vi "SW_Set_Add_Recording_Settings.vi"(2 "Offsets, swaps and rotations in":T1={"Offset V."=0.0, "Offset H."=0.0, "Bridge swap"=FALSE, "Twisted neck"=FALSE, "Name prefix"="SavedTrack", "Stop at"=0.0, "\"Stop at\" enabled"=FALSE} {"Stop at" min=0.0 max=43200.0 step=60.0 format="%<%H:%M:%S>t"}) -> (0 "Offsets, swaps and rotations out":T1={"Offset V."=0.0, "Offset H."=0.0, "Bridge swap"=FALSE, "Twisted neck"=FALSE, "Name prefix"="SavedTrack", "Stop at"=0.0, "\"Stop at\" enabled"=FALSE} {"Stop at" min=0.0 max=43200.0 step=60.0 format="%<%H:%M:%S>t"})   [LabVIEW 2016]
uses:
  <vilib>/Utility/miscctls.llb/LVPointTypeDef.ctl
panel:
  out "\"Stop at\" buffer":dbl min=0.0 max=43200.0 step=60.0 format="%<%H:%M:%S>t"
  in  "Enable":bool
  in  "Bridge hor. offset":sgl min=-70 max=70 step=0.1 format="%#.1g"
  in  "Bridge swap":bool
  in  "Bridge offset":sgl min=-70 max=70 step=0.1 format="%#.1g"
  in  "Twisted neck":bool
  in  "Name Prefix":string="SavedTrack"
  in  "Stop record at":dbl=600.0 caption="Stop at" min=0.0 max=43200.0 step=60.0 format="%<%H:%M:%S>t"
  in  "Reset to defaults":bool
  in  "Exit":bool
  in  "Save Config":bool
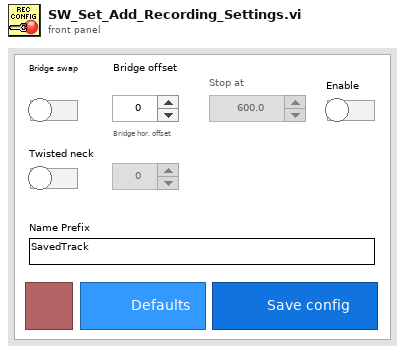
[diagram p1: front panel]
types:
  T1 = cluster{"Offset V.":sgl, "Offset H.":sgl, "Bridge swap":bool, "Twisted neck":bool, "Name prefix":string, "Stop at":dbl, "\"Stop at\" enabled":bool}
  T2 = typedef "LVPointTypeDef.ctl" = cluster{"Horizontal":i16, "Vertical":i16}
  T3 = enum8{"Enabled", "Disabled", "Disabled and Grayed Out"}
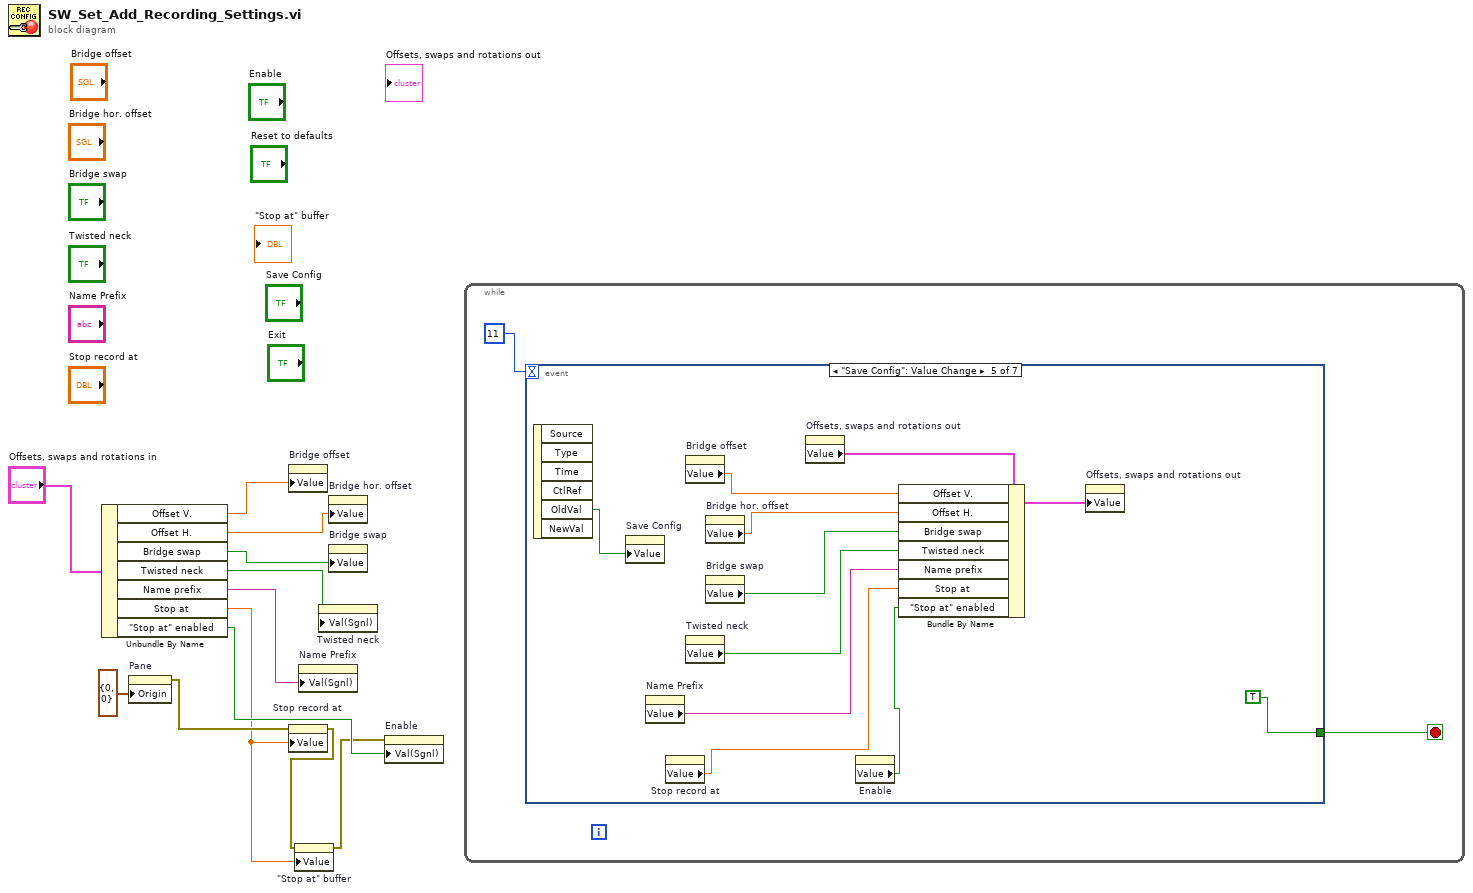
[diagram p0: block diagram]
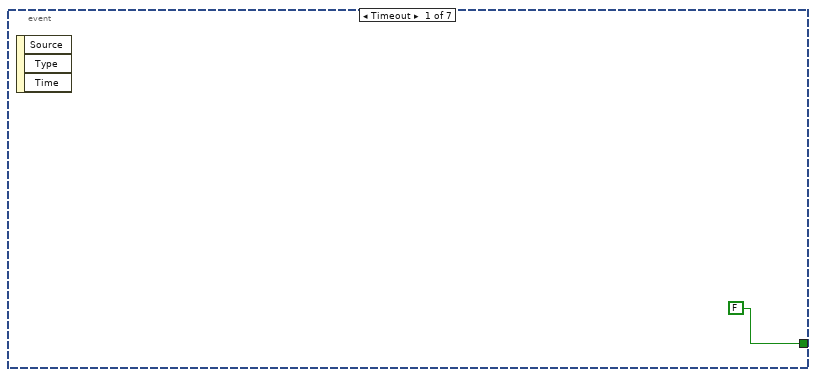
[diagram p2: hidden frame]
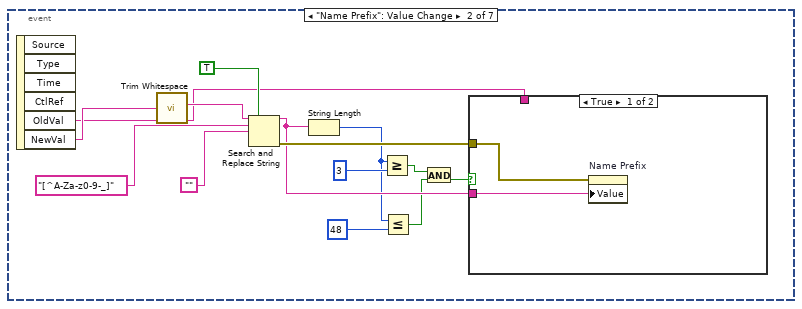
[diagram p3: hidden frame]
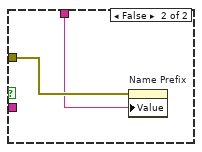
[diagram p4: hidden frame]
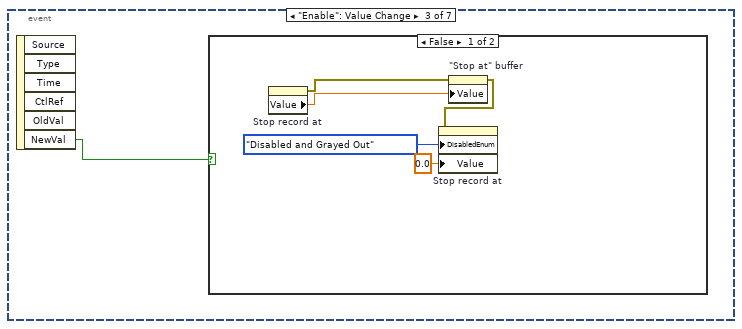
[diagram p5: hidden frame]
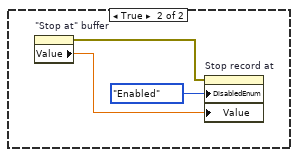
[diagram p6: hidden frame]
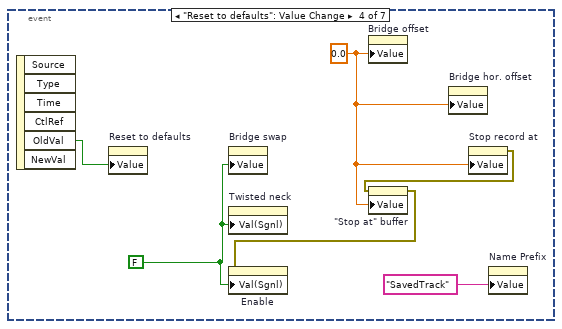
[diagram p7: hidden frame]
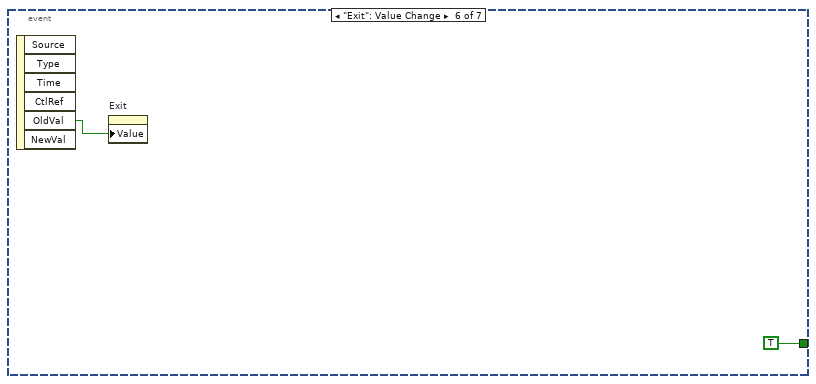
[diagram p8: hidden frame]
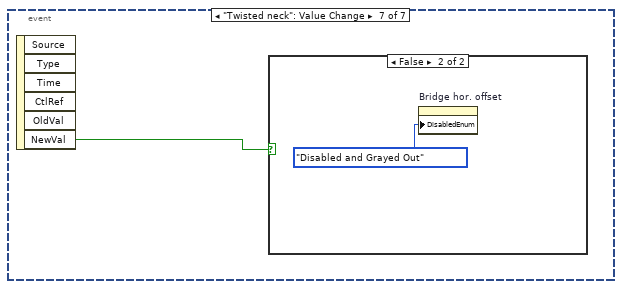
[diagram p9: hidden frame]
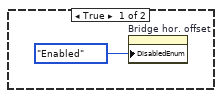
[diagram p10: hidden frame]
diagram:
  n1 = Unbundle By Name("Offsets, swaps and rotations in") -> ("Offset V."=w10:sgl, "Offset H."=w9:sgl, "Bridge swap"=w8:bool, "Twisted neck"=w7:bool, "Name prefix"=w6:string, "Stop at"=w1:dbl, "\"Stop at\" enabled"=w4:bool)
  n2 = property on="Pane" class="Pane"("Origin"=T2 {"Horizontal"=0, "Vertical"=0}) -> (error out=w5:errorcluster)  [unwired: 2 in, 1 out]
  n3 = property on="Bridge offset" class="DigNum (strict)"("Value"=w10) -> ()  [unwired: 2 in, 2 out]
  n4 = property on="Stop record at" class="DigNum (strict)"(error in=w5, "Value"=w1) -> (error out=w3:errorcluster)  [unwired: 1 in, 1 out]
  n5 = property on="\"Stop at\" buffer" class="DigNum (strict)"(error in=w3, "Value"=w1) -> (error out=w2:errorcluster)  [unwired: 1 in, 1 out]
  n6 = property on="Name Prefix" class="Str"("Val(Sgnl)"=w6) -> ()  [unwired: 2 in, 2 out]
  n7 = property on="Twisted neck" class="Bool (strict)"("Val(Sgnl)"=w7) -> ()  [unwired: 2 in, 2 out]
  n8 = property on="Bridge hor. offset" class="DigNum (strict)"("Value"=w9) -> ()  [unwired: 2 in, 2 out]
  n9 = property on="Bridge swap" class="Bool (strict)"("Value"=w8) -> ()  [unwired: 2 in, 2 out]
  n10 = property on="Enable" class="Bool (strict)"(error in=w2, "Val(Sgnl)"=w4) -> ()  [unwired: 1 in, 2 out]
  n11 = while {
    stop <- w13 stop-if-true
    n12 = event shown="[4] \"Save Config\": Value Change" {
      selector: _ -> [_ _ _ _ _ _ _]
      dyn-events: _ -> [_ _ _ _ _ _ _]
      timeout: 11 -> [_ _ _ _ _ _ _]
      tunnel: [FALSE _ _ _ TRUE TRUE _] -> w13
      event Timeout {
        n13 = event-data() -> ()  [unwired: 1 in, 3 out]
      }
      event "Name Prefix": Value Change {
        n14 = event-data() -> ("OldVal"=w20:string, "NewVal"=w21:string)  [unwired: 1 in, 4 out]
        n15 = call <vilib>:"Trim Whitespace.vi"("string"=w21) -> ("trimmed string"=w27:string)  [unwired: 1 in]
        n16 = Search and Replace String(replace all?=TRUE ("replace all? (F)"), input string=w27, search string="[^A-Za-z0-9-_]" ("regular expression"), replace string="") -> (result string=w22:string, error out=w24:errorcluster)  [unwired: 4 in, 2 out]
        n17 = String Length(string=w22) -> (length=w19:i32)
        n18 = Greater Or Equal?(x=w19, y=3) -> (x >= y?=w23:bool)
        n19 = Less Or Equal?(x=w19, y=48) -> (x <= y?=w16:bool)
        n20 = And(x=w23, y=w16) -> (x .and. y?=w17:bool)
        n21 = case shown="True" w17 {
          tunnel: w24 -> [w31 w33]
          tunnel: w22 -> [w30 _]
          tunnel: w20 -> [_ w32]
          frame True {
            n22 = property on="Name Prefix" class="Str"(error in=w31, "Value"=w30) -> ()  [unwired: 1 in, 2 out]
          }
          frame False {
            n23 = property on="Name Prefix" class="Str"(error in=w33, "Value"=w32) -> ()  [unwired: 1 in, 2 out]
          }
        }
      }
      event "Enable": Value Change {
        n24 = event-data() -> ("NewVal"=w34:bool)  [unwired: 1 in, 5 out]
        n25 = case shown="False" w34 {
          frame False {
            n26 = property on="Stop record at" class="DigNum (strict)"() -> (error out=w36:errorcluster, "Value"=w37:dbl)  [unwired: 2 in, 1 out]
            n27 = property on="\"Stop at\" buffer" class="DigNum (strict)"(error in=w36, "Value"=w37) -> (error out=w35:errorcluster)  [unwired: 1 in, 1 out]
            n28 = property on="Stop record at" class="DigNum (strict)"(error in=w35, "DisabledEnum"=T3."Disabled and Grayed Out" ("Disabled"), "Value"=0.0 ("Stop record at")) -> ()  [unwired: 1 in, 2 out]
          }
          frame True {
            n29 = property on="\"Stop at\" buffer" class="DigNum (strict)"() -> (error out=w40:errorcluster, "Value"=w41:dbl)  [unwired: 2 in, 1 out]
            n30 = property on="Stop record at" class="DigNum (strict)"(error in=w40, "DisabledEnum"=T3."Enabled" ("Disabled"), "Value"=w41) -> ()  [unwired: 1 in, 2 out]
          }
        }
      }
      event "Reset to defaults": Value Change {
        w45 = sgl 0.0 ("Bridge offset")
        w47 = FALSE
        n31 = event-data() -> ("OldVal"=w48:bool)  [unwired: 1 in, 5 out]
        n32 = property on="Reset to defaults" class="Bool (strict)"("Value"=w48) -> ()  [unwired: 2 in, 2 out]
        n33 = property on="Bridge swap" class="Bool (strict)"("Value"=w47) -> ()  [unwired: 2 in, 2 out]
        n34 = property on="Twisted neck" class="Bool (strict)"("Val(Sgnl)"=w47) -> ()  [unwired: 2 in, 2 out]
        n35 = property on="Bridge offset" class="DigNum (strict)"("Value"=w45) -> ()  [unwired: 2 in, 2 out]
        n36 = property on="Bridge hor. offset" class="DigNum (strict)"("Value"=w45) -> ()  [unwired: 2 in, 2 out]
        n37 = property on="Stop record at" class="DigNum (strict)"("Value"=w45) -> (error out=w44:errorcluster)  [unwired: 2 in, 1 out]
        n38 = property on="\"Stop at\" buffer" class="DigNum (strict)"(error in=w44, "Value"=w45) -> (error out=w43:errorcluster)  [unwired: 1 in, 1 out]
        n39 = property on="Enable" class="Bool (strict)"(error in=w43, "Val(Sgnl)"=w47) -> ()  [unwired: 1 in, 2 out]
        n40 = property on="Name Prefix" class="Str"("Value"="SavedTrack" ("Value (Signaling)")) -> ()  [unwired: 2 in, 2 out]
      }
      event "Save Config": Value Change {
        n41 = event-data() -> ("OldVal"=w56:bool)  [unwired: 1 in, 5 out]
        n42 = property on="Save Config" class="Bool (strict)"("Value"=w56) -> ()  [unwired: 2 in, 2 out]
        n43 = property on="Name Prefix" class="Str"() -> ("Value"=w51:string)  [unwired: 2 in, 2 out]
        n44 = property on="Stop record at" class="DigNum (strict)"() -> ("Value"=w50:dbl)  [unwired: 2 in, 2 out]
        n45 = property on="Bridge offset" class="DigNum (strict)"() -> ("Value"=w55:sgl)  [unwired: 2 in, 2 out]
        n46 = property on="Twisted neck" class="Bool (strict)"() -> ("Value"=w52:bool)  [unwired: 2 in, 2 out]
        n47 = property on="Bridge hor. offset" class="DigNum (strict)"() -> ("Value"=w54:sgl)  [unwired: 2 in, 2 out]
        n48 = property on="Bridge swap" class="Bool (strict)"() -> ("Value"=w53:bool)  [unwired: 2 in, 2 out]
        n49 = property on="Offsets, swaps and rotations out" class="Clust (strict)"() -> ("Value"=w58:T1)  [unwired: 2 in, 2 out]
        n50 = property on="Enable" class="Bool (strict)"() -> ("Value"=w49:bool)  [unwired: 2 in, 2 out]
        n51 = Bundle By Name(cluster=w58, "Offset V."=w55, "Offset H."=w54, "Bridge swap"=w53, "Twisted neck"=w52, "Name prefix"=w51, "Stop at"=w50, "\"Stop at\" enabled"=w49) -> (w57:T1)
        n52 = property on="Offsets, swaps and rotations out" class="Clust (strict)"("Value"=w57) -> ()  [unwired: 2 in, 2 out]
      }
      event "Exit": Value Change {
        n53 = event-data() -> ("OldVal"=w61:bool)  [unwired: 1 in, 5 out]
        n54 = property on="Exit" class="Bool (strict)"("Value"=w61) -> ()  [unwired: 2 in, 2 out]
      }
      event "Twisted neck": Value Change {
        n55 = event-data() -> ("NewVal"=w62:bool)  [unwired: 1 in, 5 out]
        n56 = case shown="False" w62 {
          frame True {
            n57 = property on="Bridge hor. offset" class="DigNum (strict)"("DisabledEnum"=T3."Enabled" ("Disabled")) -> ()  [unwired: 2 in, 2 out]
          }
          frame False {
            n58 = property on="Bridge hor. offset" class="DigNum (strict)"("DisabledEnum"=T3."Disabled and Grayed Out" ("Disabled")) -> ()  [unwired: 2 in, 2 out]
          }
        }
      }
    }
  }
